vi "Review Recipe for Overlap2.vi"(6 "Waypoints":cluster{"x":dbl, "y":dbl, "th":dbl}[](array[cluster]), 8 "Blends":T1[](array[typedef])) -> (0 "Blends out":T1[](array[typedef]), 2 "Linear Info":T2(array[cluster]), 3 "Length (f)":dbl, 4 "Waypoints out":cluster{"x":dbl, "y":dbl, "th":dbl}[](array[cluster]), 5 "Array":cluster{"x":dbl, "y":dbl, "th":dbl}[](array[cluster]))   [LabVIEW 2023]
uses:
  BlendType.ctl
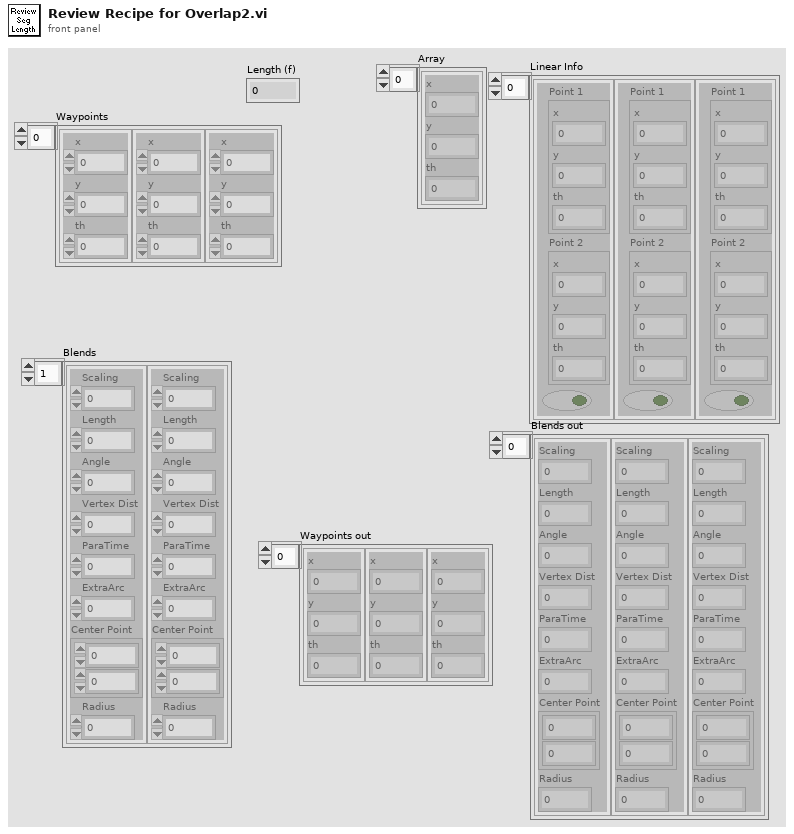
[diagram p1: front panel]
types:
  T1 = typedef "BlendType.ctl" = cluster{"Scaling":dbl, "Length":dbl, "Angle":dbl, "Vertex Dist":dbl, "ParaTime":dbl, "ExtraArc":dbl, "Center Point":cluster{dbl, dbl}, "Radius":dbl}
  T2 = cluster{"Point 1":cluster{"x":dbl, "y":dbl, "th":dbl}, "Point 2":cluster{"x":dbl, "y":dbl, "th":dbl}, bool}[]
  T3 = cluster{"Point Out":cluster{"x":dbl, "y":dbl, "th":dbl}, "Point Out":cluster{"x":dbl, "y":dbl, "th":dbl}, bool}
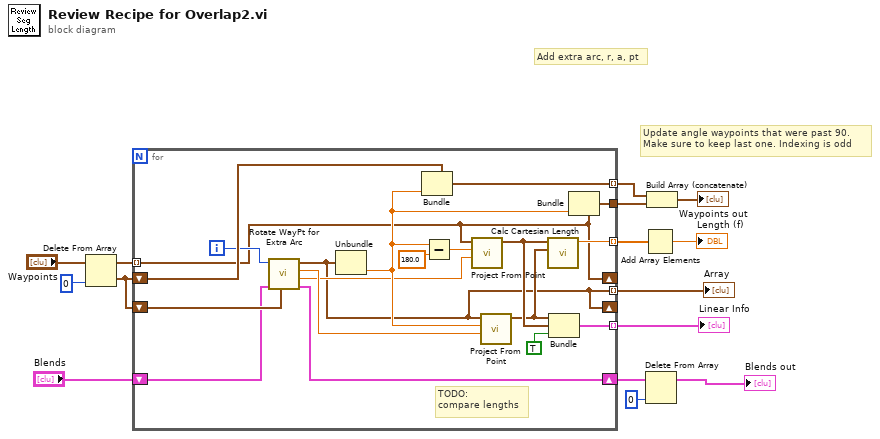
[diagram p0: block diagram]
diagram:
  # "Update angle waypoints that were past 90.\nMake sure to keep last one. Indexing is odd"
  # "Add extra arc, r, a, pt"
  n1 = Delete From Array(array="Waypoints", index=0) -> (deleted portion=w2:cluster{"x":dbl, "y":dbl, "th":dbl}, array with subset deleted=w12:cluster{"x":dbl, "y":dbl, "th":dbl}[])  [unwired: 1 in]
  n2 = for {
    tunnel: w12 -> [w16] mode=indexing
    shift-right: [w16] -> _
    shift-left: w2 -> [w27]
    tunnel: [w34] -> w13 mode=indexing
    tunnel: [w29] -> w14 mode=indexing
    tunnel: [w26] -> w6 mode=indexing
    tunnel: [w24] -> w4
    tunnel: [w17] -> w3 mode=indexing
    shift-right: [w17] -> _
    shift-left: w2 -> [w23]
    shift-right: [w20] -> w8
    shift-left: "Blends" -> [w21]
    i -> [w22]
    # "TODO:\ncompare lengths"
    n3 = call "Rotate WayPt for Extra Arc.vi"("Pt 0"=w23, "Blends In"=w21, "index"=w22) -> ("Blends Out"=w20:T1[], "Pt2 vertex dist"=w18:dbl, "Pt0 vertex dist"=w19:dbl, "Pt Out"=w17:cluster{"x":dbl, "y":dbl, "th":dbl})  [unwired: 5 in]
    n4 = Unbundle(w17) -> ("th"=w25:dbl)  [unwired: 2 out]
    n5 = Bundle(cluster=w27, "th"=w25) -> (w26:cluster{"x":dbl, "y":dbl, "th":dbl})  [unwired: 2 in]
    n6 = Subtract(x=w25, y=180.0) -> (x-y=w33:dbl)
    n7 = call "Project From Point.vi"("distance"=w18, "th"=w33, "Point In"=w16) -> ("Point Out"=w31:cluster{"x":dbl, "y":dbl, "th":dbl})  [unwired: 8 in]
    n8 = call "Project From Point.vi"("distance"=w19, "th"=w25, "Point In"=w17) -> ("Point Out"=w30:cluster{"x":dbl, "y":dbl, "th":dbl})  [unwired: 8 in]
    n9 = call "Calc Cartesian Length.vi"("Point 2"=w30, "Point 1"=w31) -> ("Length (f)"=w29:dbl)  [unwired: 8 in, 1 out]
    n10 = Bundle("Point Out"=w30, "Point Out"=w31, TRUE) -> (w34:T3)  [unwired: 1 in]
    n11 = Bundle(cluster=w16, "th"=w25) -> (w24:cluster{"x":dbl, "y":dbl, "th":dbl})  [unwired: 2 in]
  }
  "Linear Info" <- w13
  "Array" <- w3
  n12 = Add Array Elements(numeric array=w14) -> (sum=→"Length (f)":dbl)
  n13 = Delete From Array(array=w8, index=0) -> (array with subset deleted=→"Blends out":T1[])  [unwired: 1 in, 1 out]
  n14 = Build Array (concatenate)(w6, w4) -> (→"Waypoints out":cluster{"x":dbl, "y":dbl, "th":dbl}[])
